vi "Build I2C Linux.vi"(9 "Payload":u8[](array[numeric])=[10, 11, 10, 13, 11, 10, 11, 14] format="%.0x", 10 "I2C Metadata":T1={"TAI Time (ns)"=0, "7 bit Address"=0, "Bus"=0, "Read"=TRUE} {"7 bit Address" format="%.0x"}, 11 "pcap Parse and Build in":refnum<class "pcap_Parse_Build_CIF.lvclass">) -> (2 "I2C Packet":u8[](array[numeric])=[231, 76, 198, 103, 241, 40, 73, 51, 14, 0, 0, 0, 14, 0, 0, 0, 2, 0, 0, 0, 0, 128, 10, 11, 10, 13, 11, 10, 11, 14] format="%.0x", 3 "pcap Parse and Build out":refnum<class "pcap_Parse_Build_CIF.lvclass">)   [LabVIEW 2021, in "pcap_Parse_Build_CIF.lvclass"]
uses:
  pcap_Parse_Build_CIF.lvclass
  Typedef/Format Specific/I2C Metadata.ctl
  Typedef/Format Specific/I2C Linux Header.ctl
  pcap_Parse_Build_CIF.lvclass/pcap_Parse_Build_CIF.ctl
  Build/SubVIs/Flatten Packet Header.vi
  <vilib>/CIF Foundation/CIF Utilities/DataTypes/Flatten U32.vi
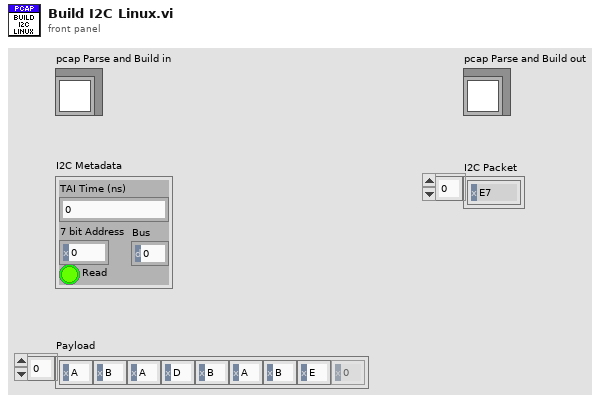
[diagram p1: front panel]
types:
  T1 = typedef "pcap_Parse_Build_CIF.lvclass/I2C Metadata.ctl" = cluster{"TAI Time (ns)":i64, "7 bit Address":u8, "Bus":u8, "Read":bool}
  T2 = typedef "pcap_Parse_Build_CIF.lvclass/I2C Linux Header.ctl" = cluster{"Bus Number and Event Flag":u8, "Flags":u32, "HW Address":u8}
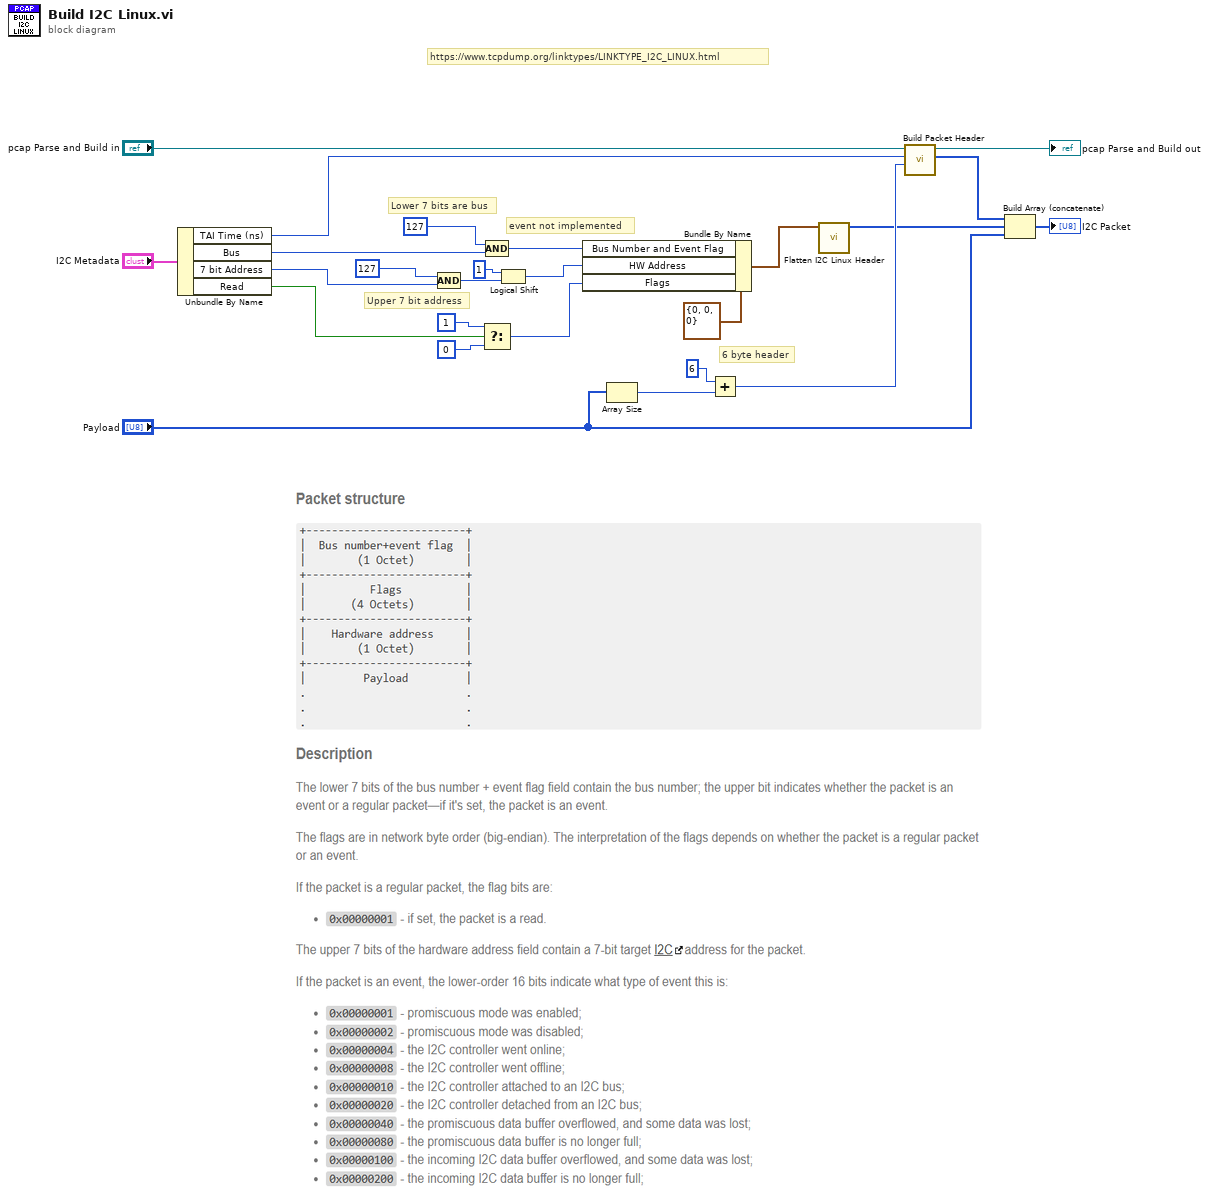
[diagram p0: block diagram]
diagram:
  # "event not implemented"
  # "Upper 7 bit address"
  # "https://www.tcpdump.org/linktypes/LINKTYPE_I2C_LINUX.html"
  # "6 byte header"
  # "Lower 7 bits are bus"
  n1 = Unbundle By Name("I2C Metadata") -> ("TAI Time (ns)"=w4:i64, "Bus"=w3:u8, "7 bit Address"=w2:u8, "Read"=w1:bool)
  n2 = Compound Arithmetic op=AND(u8 127, w2) -> (w12:u8)
  n3 = Select(t=u32 1, s=w1, f=u32 0) -> (s? t:f=w13:u32)
  n4 = Compound Arithmetic op=AND(u8 127, w3) -> (w16:u8)
  n5 = Logical Shift(y=i16 1, x=w12) -> (x << y=w11:u8)
  n6 = Bundle By Name(cluster=T2 {"Bus Number and Event Flag"=0, "Flags"=0, "HW Address"=0} ("I2C Linux Header in 2"), "Bus Number and Event Flag"=w16, "HW Address"=w11, "Flags"=w13) -> (w8:T2)
  n7 = Array Size(array="Payload") -> (size(s)=w19:i32)
  n8 = Add(x=6, y=w19) -> (x+y=w23:i32)
  n9 = call "Flatten I2C Linux Header.vi"("I2C Linux Header in"=w8) -> ("Flattened Data out"=w7:u8[])  [unwired: 10 in]
  n10 = call "Build Packet Header.vi"("Length"=w23, "TAI Time (ns)"=w4, "pcap Parse and Build in"="pcap Parse and Build in") -> ("Flattened Data out"=w22:u8[], "pcap Parse and Build out"=→"pcap Parse and Build out":refnum<class "pcap_Parse_Build_CIF.lvclass">)  [unwired: 7 in]
  n11 = Build Array (concatenate)(w22, w7, "Payload") -> (→"I2C Packet":u8[])
